vi "Parallel Loops.vi"() -> ()   [LabVIEW 2016]
panel:
  out "Loops":i32
  in  "stop":bool
  out "Step":string
  out "Shoot":bool
  out "Motor":dbl
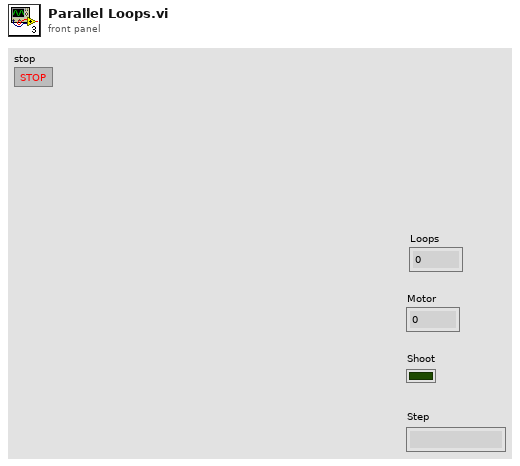
[diagram p1: front panel]
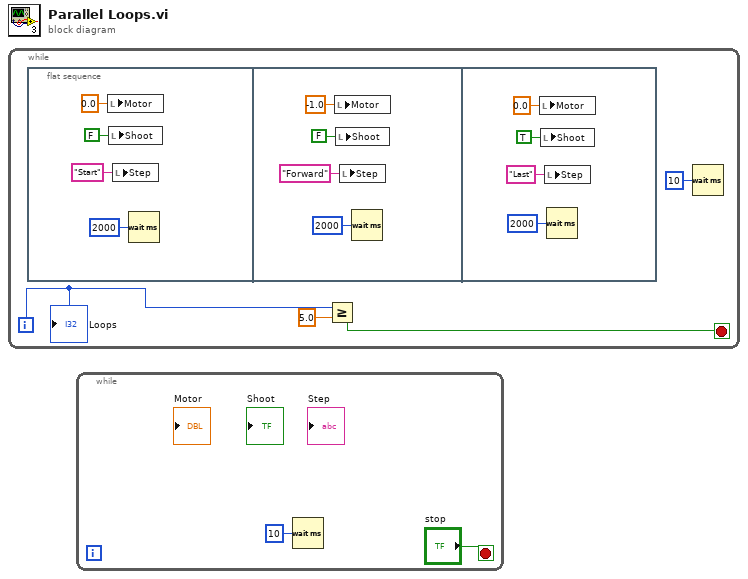
[diagram p0: block diagram]
diagram:
  n1 = while {
    i -> [w2]
    stop <- w3 stop-if-true
    n2 = flat-sequence {
      frame #0 {
        n3 = local write "Motor"(0.0 ("Motor")) -> ()
        n4 = local write "Shoot"(FALSE ("Shoot")) -> ()
        n5 = local write "Step"("Start" ("Step")) -> ()
        n6 = Wait (ms)(milliseconds to wait=u32 2000) -> ()  [unwired: 1 out]
      }
      frame #1 {
        n7 = local write "Motor"(-1.0 ("Motor")) -> ()
        n8 = local write "Shoot"(FALSE ("Shoot")) -> ()
        n9 = local write "Step"("Forward" ("Step")) -> ()
        n10 = Wait (ms)(milliseconds to wait=u32 2000) -> ()  [unwired: 1 out]
      }
      frame #2 {
        n11 = local write "Motor"(0.0 ("Motor")) -> ()
        n12 = local write "Shoot"(TRUE ("Shoot")) -> ()
        n13 = local write "Step"("Last" ("Step")) -> ()
        n14 = Wait (ms)(milliseconds to wait=u32 2000) -> ()  [unwired: 1 out]
      }
    }
    n15 = Greater Or Equal?(x=w2, y=5.0) -> (x >= y?=w3:bool)
    n16 = Wait (ms)(milliseconds to wait=u32 10) -> ()  [unwired: 1 out]
    "Loops" <- w2
  }
  n17 = while {
    stop <- "stop" stop-if-true
    n18 = Wait (ms)(milliseconds to wait=u32 10) -> ()  [unwired: 1 out]
  }
